vi "Get All Event Info.vi"(8 "First T0":timestamp, 9 "Array Size":i32, 10 "CSV Settings":T1, 11 "Tdms File Ref In":refnum<k34>) -> (3 "Test Info Column Data":string[][](array[string]))   [LabVIEW 2022 SP3, in "CSV Export.lvlib" / "CSV Export.lvclass"]
uses:
  CSV Export.lvclass
  Controls/CSV Export Settings.ctl
  CSV Export.lvclass/CSV Export.ctl
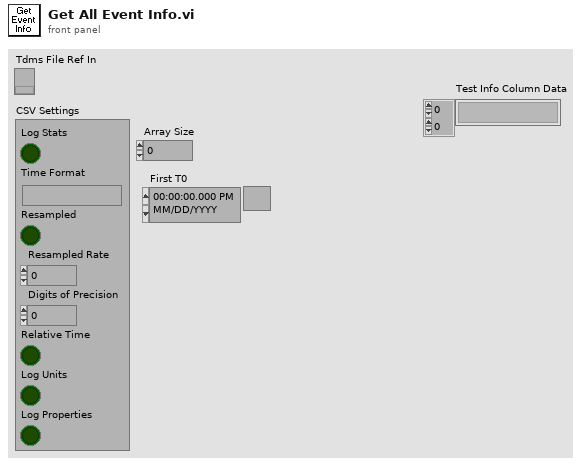
[diagram p1: front panel]
types:
  T1 = typedef "CSV Export.lvlib/CSV Export.lvclass/CSV Export Settings.ctl" = cluster{"Log Stats":bool, "Time Format":string, "Resampled":bool, "Resampled Rate":dbl, "Digits of Precision":u32, "Relative Time":bool, "Log Units":bool, "Log Properties":bool}
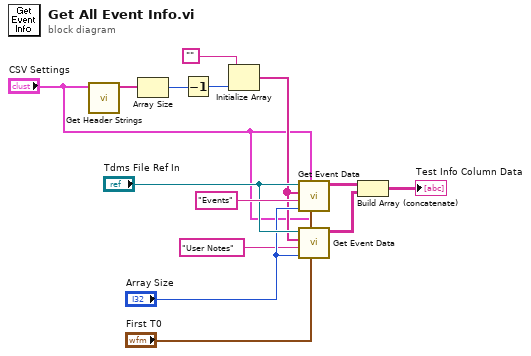
[diagram p0: block diagram]
diagram:
  n1 = call "Get Header Strings.vi"("CSV Settings"="CSV Settings") -> ("Header Values"=w14:string[])  [unwired: 10 in]
  n2 = Array Size(array=w14) -> (size(s)=w13:i32)
  n3 = Decrement(x=w13) -> (x-1=w12:i32)
  n4 = Initialize Array("", w12) -> (w7:string[])
  n5 = call "Get Event Data.vi"("First T0"="First T0", "CSV Settings"="CSV Settings", "Array Size"="Array Size", "group name"="Events", "Header padding"=w7, "Refnum in"="Tdms File Ref In") -> ("Array out"=w5:string[][])  [unwired: 5 in]
  n6 = call "Get Event Data.vi"("First T0"="First T0", "CSV Settings"="CSV Settings", "Array Size"="Array Size", "group name"="User Notes", "Header padding"=w7, "Refnum in"="Tdms File Ref In") -> ("Array out"=w4:string[][])  [unwired: 5 in]
  n7 = Build Array (concatenate)(w5, w4) -> (→"Test Info Column Data":string[][])
